vi "myVelocimeter_(Please use Run, not Open).vi"() -> ()   [LabVIEW 2018]
doc: "This is the main VI of the myVelocimeter program. It provides user with ability to calculate the acceleration due to gravity by performing calculations based on the input method that is user defined. User has a choice of performing the test using myDAQ (or similar) equipment or run the simulation based on the data file provided.\n\nThe actual test was design to obtain the value of acceleration due to gravity using myDAQ (or similar) equipment, light gate detector, encoder wheel (fine adjustments and settings available to cater for use with various equimpent) with thread on its axle and weight attached to it.\n\nTo perform the test once the actual encoder wheel details are adjusted, the 'Run Test' option needs to be selected upon first prompt. This then starts the test and program is already aquiring the data. At this point the weight must be dropped and program will display all data it is aquiring and proccesing in real time. Once the thread is fully unwinded, program will automatically stop and provide the value of acceleration due to gravity. At this point, the program will prompt user whether to save the data acquired and then to either run another test or end the program.\n\nThe simulation mode is also available. This mode require a data file with time and encoder counts values to mimic the actual test. The outcome is exactly the same as the one from the actual test. Once all data is processed, the program will prompt user whether to save the data acquired and then to either run another test or end the program.\n\nThe program was design to acquire data and process it in real time with equipment such as myDAQ with ability to save all this data to a file. This file can then be run in a simulation mode to recreate the actual test without the need of any physically devices.\n\nInputs:\nDevice + Encoder Channel;\nAxle Radius (m);\nNumber Of Slits;\nError In.\n\nOutputs:\nEncoder Counts;\nNumber Of Rotations;\nCurrent Rotary Speed (rad/s);\nCurrent Linear Speed (m/s);\nLinear Distance (m);\nCurrent Time (s);\nAcceleration due to gravity (m/s^2);\nSave File;\nSave File To;\nArray;\nSpeed vs Time Graph;\nMaximum Linear Speed (m/s) and Time Occured (s);\nMinimum Linear Speed (m/s) and Time Occured (s);\nError Out."
uses:
  Type Defs/States.ctl
  <vilib>/DAQmx/read.llb/DAQmx Read (Counter DBL 1Chan 1Samp).vi
  <vilib>/DAQmx/miscellaneous.llb/DAQmx Fill In Error Info.vi
panel:
  in  "Stop Test":bool
  in  "Begin Test":bool
  in  "Main Settings":T1={"Device + Encoder Channel"="myDAQ1/ctr0", "Axle Radius (m)"=0.0042, "No of Slits"=4.0} {"Axle Radius (m)" format="%#_13g"}
  out "Min/Max Linear Speed":T2 {"Maximum Linear Speed (m/s)" format="%#_2g"}
  out "File Saved?":bool
  out "Save File To":path
  out "error out":errorcluster
  in  "error in":errorcluster
  out "Data Stored":dbl[][](array[numeric]) format="%.2f"
  out "Linear Speed vs Time Graph":cluster{"Y":dbl[], "Y":dbl[]}[](graph)
  in  "Exit Program":bool
  out "Output Data":T3 {"Acceleration due to Gravity (m/s^2)" format="%#.2g"; "Current Time (s)" format="%#.2g"; "Current Rotary Speed (rad/s)" format="%#.2g"; "Linear Distance (m)" format="%#.2g"; "Current Linear Speed (m/s)" format="%#.2g"}
  # "No. of \nRotations"
  # "Current Rotary\nSpeed (rad/s)"
  # "Linear\nDistance (m)"
  # "Current Linear\nSpeed (m/s)"
  # "Time (s)"
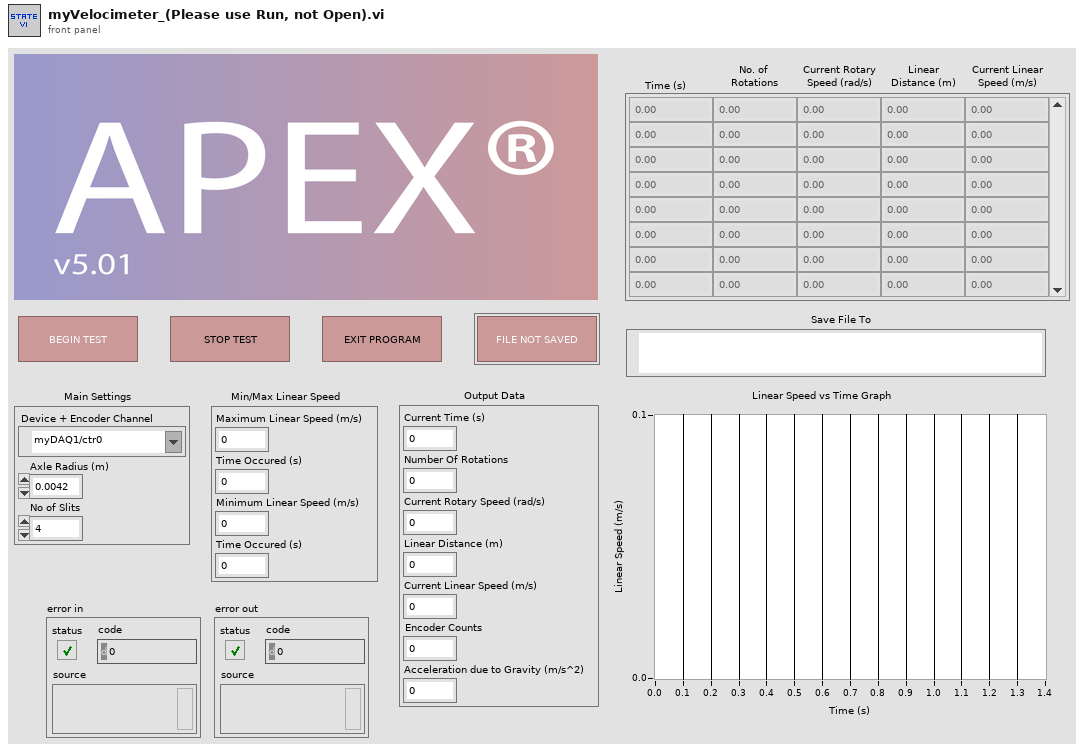
[diagram p1: front panel]
types:
  T1 = cluster{"Device + Encoder Channel":tag, "Axle Radius (m)":dbl, "No of Slits":dbl}
  T2 = cluster{"Maximum Linear Speed (m/s)":dbl, "Time Occured (s)":dbl, "Minimum Linear Speed (m/s)":dbl, "Time Occured (s)":dbl}
  T3 = cluster{"Current Time (s)":dbl, "Number Of Rotations":dbl, "Current Rotary Speed (rad/s)":dbl, "Linear Distance (m)":dbl, "Current Linear Speed (m/s)":dbl, "Encoder Counts":dbl, "Acceleration due to Gravity (m/s^2)":dbl}
  T4 = typedef "States.ctl" = enum16{"Idle", "Initialise", "Select Method", "Process Data", "End"}
  T5 = cluster{dbl[], "Current Linear Speed (m/s)":dbl, "Axle Radius (m)":dbl, "Current Linear Speed (m/s)":dbl, "No of Slits":dbl, "data":dbl, "Current Linear Speed (m/s)":dbl}
  T6 = cluster{"Change In Linear Distance":dbl, "Array":dbl[], "Current Linear Speed (m/s)":dbl, "Acceleration due to gravity (m/s^2)":dbl, "Number Of Rotations":dbl, "Current Rotary Speed":dbl, "Linear Distance":dbl}
  T7 = cluster{"Current Linear Speed (m/s)":dbl, "Current Rotary Speed":dbl}
  T8 = cluster{"Current Linear Speed (m/s)":dbl, "Number Of Rotations":dbl, "Current Rotary Speed":dbl, "Linear Distance":dbl, "Current Linear Speed (m/s)":dbl, "data":dbl, "Acceleration due to gravity (m/s^2)":dbl}
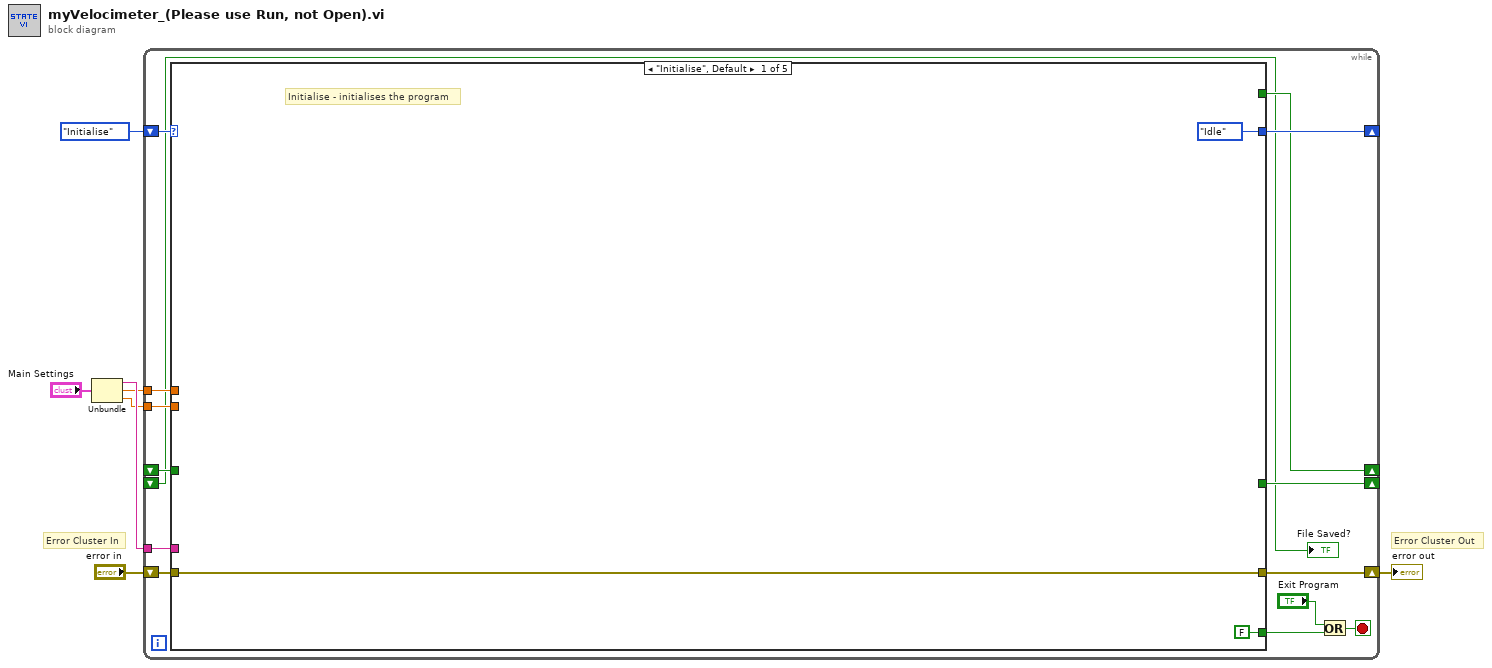
[diagram p0: block diagram]
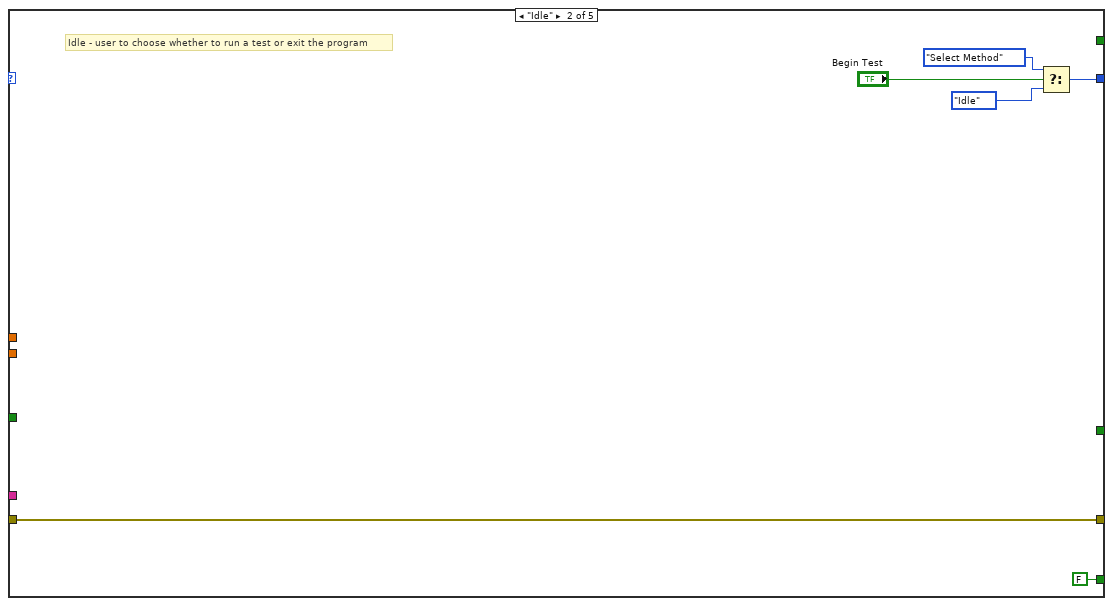
[diagram p2: hidden frame]
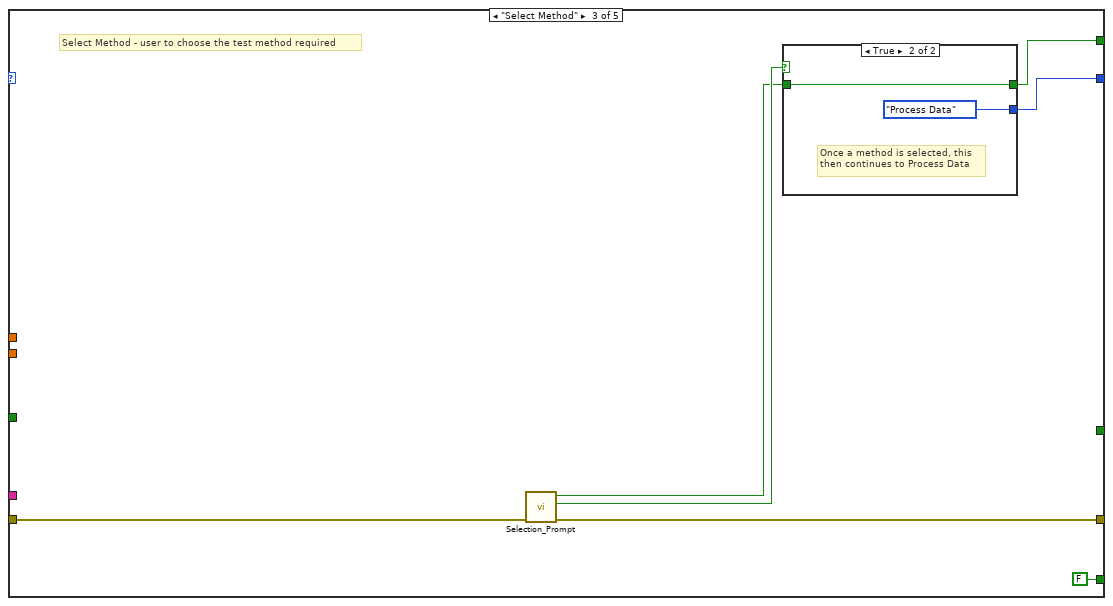
[diagram p3: hidden frame]
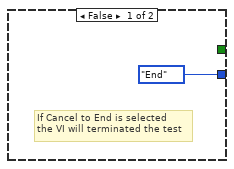
[diagram p4: hidden frame]
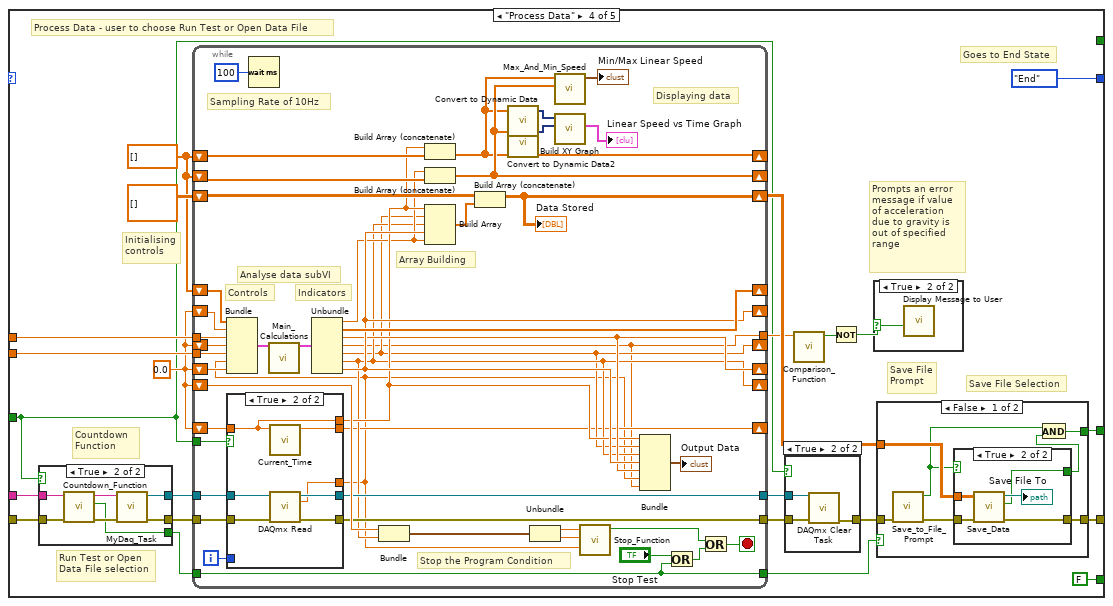
[diagram p5: hidden frame]
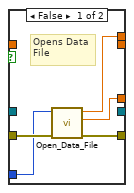
[diagram p11: hidden frame]
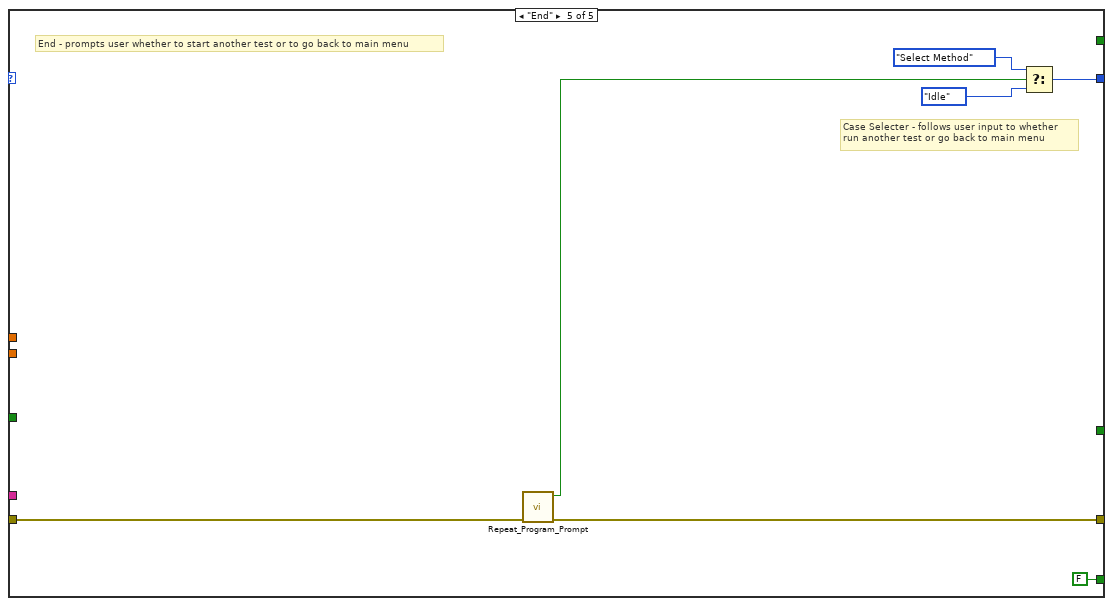
[diagram p12: hidden frame]
diagram:
  # "Error Cluster Out"
  # "Error Cluster In"
  n1 = Unbundle("Main Settings") -> ("Device + Encoder Channel"=w3:tag, "Axle Radius (m)"=w2:dbl, "No of Slits"=w1:dbl)
  n2 = while {
    shift-right: [w21] -> _
    shift-left: States."Initialise" -> [w19]
    shift-right: [w18] -> w5
    shift-left: "error in" -> [w20]
    shift-right: [w17] -> _
    shift-left: _ -> [w16]
    tunnel: w2 -> [w15]
    tunnel: w1 -> [w14]
    tunnel: w3 -> [w13]
    shift-right: [w9] -> _
    shift-left: _ -> [w8]
    stop <- w12 stop-if-true
    n3 = case shown="\"Initialise\", Default" w19 {
      tunnel: [States."Idle" w28 w33 States."End" w152] -> w21
      tunnel: w20 -> [w23 w30 w37 w60 w155]
      tunnel: [w23 w30 w36 w61 w154] -> w18
      tunnel: [FALSE ("False") FALSE ("False") FALSE ("False") FALSE ("False") FALSE ("False")] -> w11
      tunnel: [_ _ w32 _ _] -> w17
      tunnel: w16 -> [_ _ _ w41 _]
      tunnel: w15 -> [_ _ _ w55 _]
      tunnel: w14 -> [_ _ _ w54 _]
      tunnel: w13 -> [_ _ _ w49 _]
      tunnel: [_ _ _ w43 _] -> w9
      frame "Initialise", Default {
        # "Initialise - initialises the program"
      }
      frame "Idle" {
        # "Idle - user to choose whether to run a test or exit the program"
        n4 = Select(t=States."Select Method", s="Begin Test", f=States."Idle") -> (s? t:f=w28:T4)
      }
      frame "Select Method" {
        # "Select Method - user to choose the test method required"
        n5 = call "Selection_Prompt.vi"("error in (no error)"=w37) -> ("error out"=w36:errorcluster, "OK"=w35:bool, "Collect Data"=w34:bool)  [unwired: 8 in]
        n6 = case shown="True" w35 {
          tunnel: w34 -> [_ w40]
          tunnel: [States."End" States."Process Data"] -> w33
          tunnel: [_ w40] -> w32
          frame False {
            # "If Cancel to End is selected\nthe VI will terminated the test"
          }
          frame True {
            # "Once a method is selected, this\nthen continues to Process Data"
          }
        }
      }
      frame "Process Data" {
        w48 = 0.0 ("Current Linear Speed (m/s)")
        w46 = dbl[] []
        # "Save File\nPrompt"
        # "Save File Selection"
        # "Countdown\nFunction"
        # "Prompts an error \nmessage if value \nof acceleration\ndue to gravity is\nout of specified\nrange"
        # "Process Data - user to choose Run Test or Open Data File"
        # "Initialising\ncontrols"
        # "Run Test or Open\nData File selection"
        # "Goes to End State"
        n7 = case shown="True" w41 {
          tunnel: w60 -> [w83 w86]
          tunnel: [w83 w88] -> w47
          tunnel: [_ w89] -> w59
          tunnel: w49 -> [_ w87]
          tunnel: [_ w84] -> w45
          frame False {
          }
          frame True {
            n8 = call "Countdown_Function.vi"("error in (no error)"=w86) -> ("error out"=w85:errorcluster, "Stop?"=w84:bool)  [unwired: 9 in]
            n9 = call "MyDaq_Task.vi"("error in (no error)"=w85, "Device + Encoder Channel"=w87) -> ("error out"=w88:errorcluster, "Refnum out"=w89:refnum<k21>)  [unwired: 8 in]
          }
        }
        n10 = while {
          shift-right: [w98] -> w53
          shift-left: dbl[][] [] -> [w128]
          shift-right: [w123] -> _
          shift-left: w46 -> [w136]
          shift-right: [w125] -> _
          shift-left: w46 -> [w126]
          shift-right: [w97] -> _
          shift-left: w48 -> [w109]
          shift-right: [w105] -> _
          shift-left: w48 -> [w111]
          shift-right: [w99] -> _
          shift-left: w48 -> [w122]
          tunnel: [w120] -> w57
          shift-right: [w103] -> _
          shift-left: w48 -> [w107]
          shift-right: [w106] -> _
          shift-left: w46 -> [w112]
          tunnel: w47 -> [w117]
          tunnel: w41 -> [w116]
          tunnel: w59 -> [w115]
          tunnel: [w114] -> w58
          shift-right: [w96] -> _
          shift-left: w48 -> [w113]
          tunnel: [w93] -> w52
          tunnel: w55 -> [w110]
          tunnel: w54 -> [w108]
          tunnel: w45 -> [w90]
          tunnel: [w90] -> w44
          i -> [w119]
          stop <- w121 stop-if-true
          # "Analyse data subVI"
          # "Displaying data"
          # "Stop the Program Condition"
          # "Array Building"
          # "Sampling Rate of 10Hz"
          # "Indicators"
          # "Controls"
          n11 = case shown="True" w116 {
            tunnel: [w141 w147] -> w120
            tunnel: w119 -> [w137 _]
            tunnel: [w140 w145] -> w94
            tunnel: [w139 w143] -> w101
            tunnel: w117 -> [w138 w142]
            tunnel: w115 -> [_ w148]
            tunnel: [_ w146] -> w114
            tunnel: [_ w144] -> w96
            tunnel: w113 -> [_ w143]
            frame False {
              # "Opens Data\nFile"
              n12 = call "Open_Data_File.vi"("error in (no error)"=w138, "Number of Iterations"=w137) -> ("error out"=w141:errorcluster, "Encoder Counts"=w140:dbl, "Time"=w139:dbl)  [unwired: 7 in]
            }
            frame True {
              n13 = call "Current_Time.vi"("Current Time prev"=w143) -> ("Current Time"=w144:dbl)  [unwired: 10 in]
              n14 = call-poly <vilib>:"DAQmx Read.vi"("task/channels in"=w148, "error in"=w142) -> ("task out"=w146:refnum<k21>, "data"=w145:dbl, "error out"=w147:errorcluster)  [unwired: 11 in]
            }
          }
          n15 = Bundle(w112, "Current Linear Speed (m/s)"=w111, "Axle Radius (m)"=w110, "Current Linear Speed (m/s)"=w109, "No of Slits"=w108, "data"=w94, "Current Linear Speed (m/s)"=w107) -> (w104:T5)  [unwired: 1 in]
          n16 = Wait (ms)(milliseconds to wait=u32 100) -> ()  [unwired: 1 out]
          n17 = call "Main_Calculations.vi"("Controls"=w104) -> ("Indicators"=w102:T6)  [unwired: 14 in]
          n18 = Unbundle(w102) -> ("Change In Linear Distance"=w100:dbl, "Array"=w106:dbl[], "Current Linear Speed (m/s)"=w103:dbl, "Acceleration due to gravity (m/s^2)"=w93:dbl, "Number Of Rotations"=w97:dbl, "Current Rotary Speed"=w99:dbl, "Linear Distance"=w105:dbl)
          n19 = Bundle("Current Linear Speed (m/s)"=w122, "Current Rotary Speed"=w99) -> (w131:T7)  [unwired: 1 in]
          n20 = Build Array (concatenate)(w101, w136) -> (w123:dbl[])
          n21 = Build Array (concatenate)(w100, w126) -> (w125:dbl[])
          n22 = Build Array(w101, w97, w99, w105, w100) -> (w127:dbl[])
          n23 = Build Array (concatenate)(w128, w127) -> (w98:dbl[][])
          "Data Stored" <- w98
          n24 = call "Convert to Dynamic Data"("Array"=w123) -> ("Dynamic Data Type"=w135:dynamicdata)  [unwired: 3 in]
          n25 = call "Convert to Dynamic Data2"("Array"=w125) -> ("Dynamic Data Type"=w134:dynamicdata)  [unwired: 3 in]
          n26 = Unbundle(w131) -> ("Current Linear Speed (m/s)"=w130:dbl, "Current Rotary Speed"=w129:dbl)
          n27 = call "Max_And_Min_Speed.vi"("Time Array"=w125, "Linear Speed Array"=w123) -> ("Min/Max Linear Speed"=→"Min/Max Linear Speed":T2)  [unwired: 9 in]
          n28 = call "Build XY Graph"("Y Input"=w134, "X Input"=w135) -> ("XY Graph"=→"Linear Speed vs Time Graph":cluster{"X":dbl[], "Y":dbl[]}[])  [unwired: 8 in, 1 out]
          n29 = call "Stop_Function.vi"("Encoder Counts"=w94, "Current Rotary Speed"=w129, "Current Rotary Speed prev"=w130) -> ("Stop"=w132:bool)  [unwired: 8 in]
          n30 = Bundle("Current Linear Speed (m/s)"=w101, "Number Of Rotations"=w97, "Current Rotary Speed"=w99, "Linear Distance"=w105, "Current Linear Speed (m/s)"=w103, "data"=w94, "Acceleration due to gravity (m/s^2)"=w93) -> (→"Output Data":T8)  [unwired: 1 in]
          n31 = Or(x="Stop Test", y=w90) -> (x .or. y?=w91:bool)
          n32 = Or(x=w132, y=w91) -> (x .or. y?=w121:bool)
        }
        n33 = case shown="True" w41 {
          tunnel: w58 -> [_ w82]
          tunnel: w57 -> [w79 w80]
          tunnel: [w79 w81] -> w56
          frame False {
          }
          frame True {
            n34 = call <vilib>:"DAQmx Clear Task.vi"("task in"=w82, "error in"=w80) -> ("error out"=w81:errorcluster)  [unwired: 13 in]
          }
        }
        n35 = call "Comparison_Function.vi"("Value of acceleration due to gravity"=w52) -> ("Within Specified Value?"=w51:bool)  [unwired: 10 in]
        n36 = Not(x=w51) -> (.not. x?=w50:bool)
        n37 = case shown="True" w50 {
          selector: w50 -> [_ w78]
          frame False {
          }
          frame True {
            n38 = call "Display Message to User"("Enable"=w78) -> ()  [unwired: 9 in, 2 out]
          }
        }
        n39 = case shown="False" w44 {
          tunnel: [w69 w77] -> w61
          tunnel: w56 -> [w68 w77]
          tunnel: w53 -> [w67 _]
          tunnel: [w64 _] -> w43
          frame False {
            n40 = call "Save_to_File_Prompt.vi"("error in (no error)"=w68) -> ("error out"=w70:errorcluster, "Yes"=w65:bool)  [unwired: 9 in]
            n41 = case shown="True" w65 {
              tunnel: w70 -> [w71 w76]
              tunnel: [w71 w75] -> w69
              tunnel: w67 -> [_ w74]
              tunnel: [_ w72] -> w66
              frame False {
              }
              frame True {
                n42 = call "Save_Data.vi"("error in (no error)"=w76, "Array"=w74) -> ("error out"=w75:errorcluster, "Boolean"=w72:bool, "Path"=→"Save File To":path)  [unwired: 7 in]
              }
            }
            n43 = And(x=w65, y=w66) -> (x .and. y?=w64:bool)
          }
          frame True {
          }
        }
      }
      frame "End" {
        # "Case Selecter - follows user input to whether\nrun another test or go back to main menu"
        # "End - prompts user whether to start another test or to go back to main menu"
        n44 = call "Repeat_Program_Prompt.vi"("error in (no error)"=w155) -> ("error out"=w154:errorcluster, "Yes"=w151:bool)  [unwired: 9 in]
        n45 = Select(t=States."Select Method", s=w151, f=States."Idle") -> (s? t:f=w152:T4)
      }
    }
    n46 = Or(x="Exit Program", y=w11) -> (x .or. y?=w12:bool)
    "File Saved?" <- w8
  }
  "error out" <- w5
